vi "COMI US Stop.vi"(10 "bReleaseBuf":i32, 11 "hDevice":u32) -> (2 "function return":i32, 3 "hDevice out":u32)   [LabVIEW 2017, in "Comidll.lvlib"]
doc: "int (COMI_US_Stop) (HANDLE hDevice, int bReleaseBuf);"
uses:
  <userlib>/Comidll/Comidll.lvlib
  <userlib>/Comidll/Comidll.dll
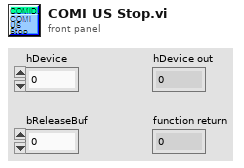
[diagram p1: front panel]
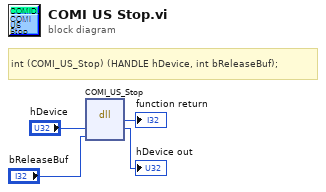
[diagram p0: block diagram]
diagram:
  # "int\t(COMI_US_Stop) (HANDLE hDevice, int bReleaseBuf);"
  n1 = dll-call lib="C:/Program Files/National Instruments/LabVIEW 2017/user.lib/Comidll/Comidll.*" fn="COMI_US_Stop"("hDevice"="hDevice", "bReleaseBuf"="bReleaseBuf") -> (→"function return":i32, "hDevice"=→"hDevice out":u32)  [unwired: 4 in, 2 out]
